vi "OA_PlotWksCols.vi"(4 "plotType":i32=200, 5 "r2":i32=-1, 6 "c2":i32=-1, 7 "r1":i32, 8 "error in (no error)":errorcluster, 9 "c1":i32, 10 "Origin.Worksheet in":refnum<k7>, 11 "Origin.GraphLayer in":refnum<k7>) -> (0 "error out":errorcluster, 1 "Origin.DataPlot":refnum<k7>, 2 "Origin.Worksheet Out":refnum<k7>, 3 "Origin.GraphLayer Out":refnum<k7>)   [LabVIEW 2010]
doc: "Plot a range from a worksheet to a graph layer. Supported plot type include\n200 = line (default)\n201 = scatter\n202 = line symbol\n230 = unknown, use template settings"
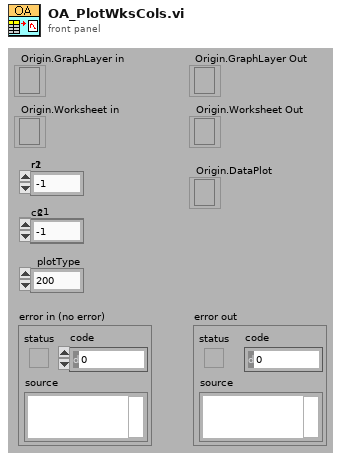
[diagram p1: front panel]
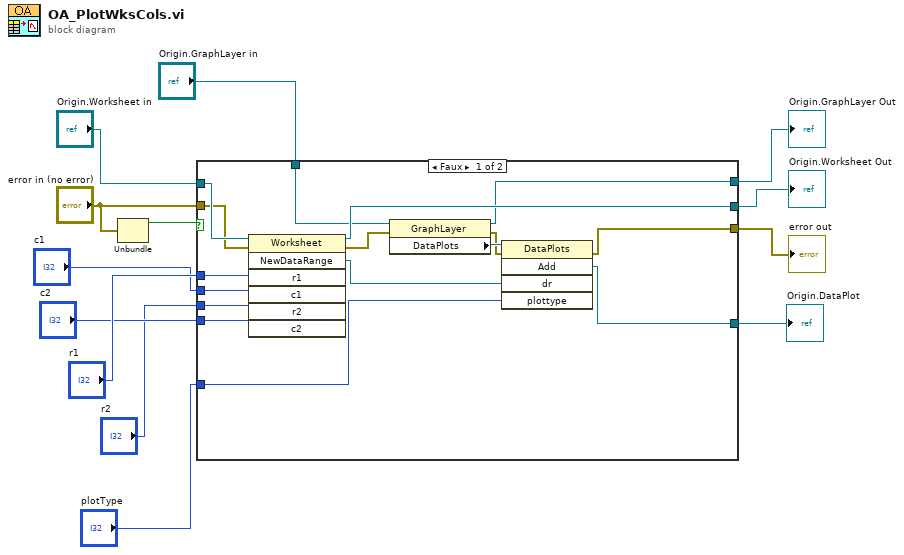
[diagram p0: block diagram]
diagram:
  n1 = Unbundle("error in (no error)") -> ("status"=w10:bool)  [unwired: 2 out]
  n2 = case shown="Faux" w10 {
    tunnel: "Origin.Worksheet in" -> [w29 w31]
    tunnel: "error in (no error)" -> [w28 w32]
    tunnel: [w15 w32] -> w12
    tunnel: "r1" -> [w27 _]
    tunnel: "c1" -> [w26 _]
    tunnel: "c2" -> [w24 _]
    tunnel: "r2" -> [w25 _]
    tunnel: "Origin.GraphLayer in" -> [w22 w30]
    tunnel: "plotType" -> [w18 _]
    tunnel: [w23 w31] -> w3
    tunnel: [w14 w30] -> w2
    tunnel: [w16 _] -> w1
    frame False {
      n3 = invoke class="Worksheet" method="NewDataRange"(reference=w29, error in=w28, "r1"=w27, "c1"=w26, "r2"=w25, "c2"=w24) -> (reference out=w23:refnum<k7>, error out=w21:errorcluster, "NewDataRange"=w17:refnum<k7>)  [unwired: 1 in, 4 out]
      n4 = property class="GraphLayer"(reference=w22, error in=w21) -> (reference out=w14:refnum<k7>, error out=w19:errorcluster, "DataPlots"=w20:refnum<k7>)
      n5 = invoke class="DataPlots" method="Add"(reference=w20, error in=w19, "dr"=w17, "plottype"=w18) -> (error out=w15:errorcluster, "Add"=w16:refnum<k7>)  [unwired: 1 in, 3 out]
    }
    frame True {
    }
  }
  "error out" <- w12
  "Origin.DataPlot" <- w1
  "Origin.Worksheet Out" <- w3
  "Origin.GraphLayer Out" <- w2
